vi "DoCreateError.vi"(5 "MergeErrors":bool, 6 "AdditionalText":string, 7 "Data":variant, 8 "ErrorIn":errorcluster caption="Error In", 9 "Text":string, 10 "ErrorCode":i32, 11 "ObjectIn":refnum<class "ErrorCreationMGI.lvclass"> caption="Object In") -> (0 "ErrorOut":errorcluster caption="Error Out", 3 "ObjectOut":refnum<class "ErrorCreationMGI.lvclass"> caption="Object Out")   [LabVIEW 2021, in "ErrorCreationMGI.lvclass"]
uses:
  ErrorCreationMGI.lvclass
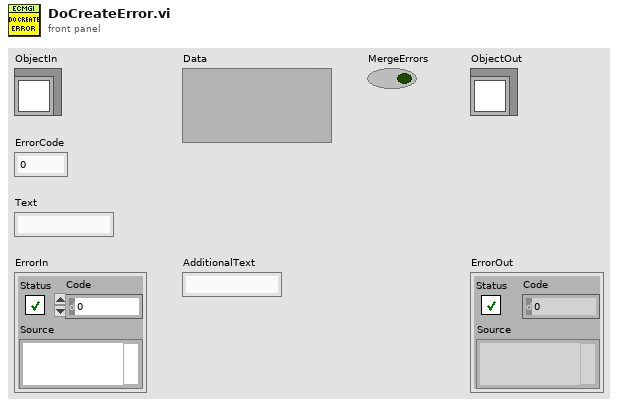
[diagram p1: front panel]
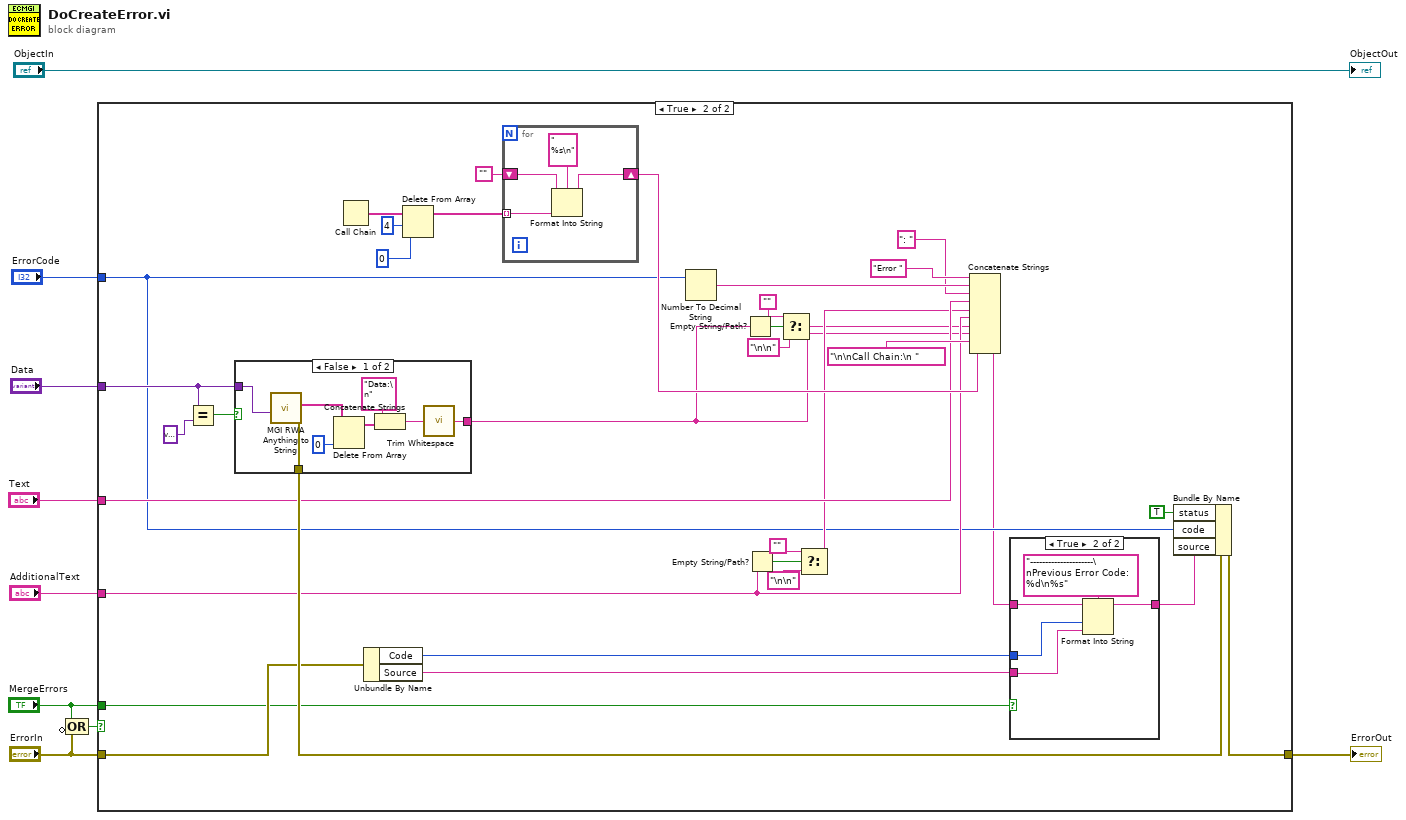
[diagram p0: block diagram]
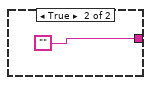
[diagram p4: hidden frame]
diagram:
  n1 = Compound Arithmetic op=OR("MergeErrors", invert "ErrorIn") -> (w3:bool)
  n2 = case shown="True" w3 {
    tunnel: "ErrorIn" -> [w10 w16]
    tunnel: [w10 w44] -> w9
    tunnel: "Data" -> [_ w43]
    tunnel: "Text" -> [_ w28]
    tunnel: "AdditionalText" -> [_ w22]
    tunnel: "ErrorCode" -> [_ w17]
    tunnel: "MergeErrors" -> [_ w15]
    frame False {
    }
    frame True {
      n3 = Equal?(x=w43, y=variant) -> (x = y?=w40:bool)
      n4 = case shown="False" w40 {
        tunnel: [w55 ""] -> w20
        tunnel: w43 -> [w58 _]
        tunnel: [w56 _] -> w39
        frame False {
          n5 = call <userlib>:"MGI RWA Anything to String.vi"("Anything"=w58) -> ("Error Out"=w56:errorcluster, "Strings[]"=w61:string[])  [unwired: 7 in, 2 out]
          n6 = Delete From Array(array=w61, index=0) -> (array with subset deleted=w62:string[])  [unwired: 1 in, 1 out]
          n7 = Concatenate Strings("Data:\n" ("string"), w62) -> (w59:string)
          n8 = call <vilib>:"Trim Whitespace.vi"("string"=w59) -> ("trimmed string"=w55:string)  [unwired: 1 in]
        }
        frame True {
        }
      }
      n9 = Call Chain() -> (call chain=w37:string[])
      n10 = Unbundle By Name(w16) -> ("Code"=w14:i32, "Source"=w13:string)
      n11 = Delete From Array(array=w37, length=4, index=0 ("length")) -> (array with subset deleted=w36:string[])  [unwired: 1 out]
      n12 = for {
        tunnel: w36 -> [w54] mode=indexing
        shift-right: [w52] -> w29
        shift-left: "" -> [w53]
        n13 = Format Into String(format string="  %s\n", initial string=w53, w54) -> (resulting string=w52:string)  [unwired: 1 in, 1 out]
      }
      n14 = Number To Decimal String(number=w17) -> (decimal integer string=w32:string)  [unwired: 1 in]
      n15 = Empty String/Path?(string/path=w20) -> (empty?=w24:bool)
      n16 = Empty String/Path?(string/path=w22) -> (empty?=w27:bool)
      n17 = Select(t="", s=w24, f="\n\n") -> (s? t:f=w21:string)
      n18 = Select(t="", s=w27, f="\n\n") -> (s? t:f=w23:string)
      n19 = Concatenate Strings("Error " ("format string"), w32, ": " ("format string"), w28, w23, w22, w21, w20, "\n\nCall Chain:\n " ("format string"), w29) -> (w12:string)
      n20 = case shown="True" w15 {
        tunnel: w14 -> [_ w47]
        tunnel: w13 -> [_ w46]
        tunnel: w12 -> [w45 w50]
        tunnel: [w45 w49] -> w11
        frame False {
        }
        frame True {
          n21 = Format Into String(format string="---------------------\nPrevious Error Code: %d\n%s", initial string=w50, w47, w46) -> (resulting string=w49:string)  [unwired: 1 in, 1 out]
        }
      }
      n22 = Bundle By Name(cluster=w39, "status"=TRUE, "code"=w17, "source"=w11) -> (w44:errorcluster)
    }
  }
  "ErrorOut" <- w9
  "ObjectOut" <- "ObjectIn"
